vi "Pump Initialize Hardware References.vi"(8 "error in (no error)":errorcluster, 11 "Hardware Resources in":T1 {"Pump Info"."Direction" items=["CW", "CCW"]; "Pump Info"."Speed" format="%03.0f"}) -> (0 "error out":errorcluster, 3 "Hardware Resources out":T1 {"Pump Info"."Direction" items=["CW", "CCW"]; "Pump Info"."Speed" format="%03.0f"})   [LabVIEW 2020, in "Pump.lvlib"]
doc: "Initialize the hardware references."
uses:
  Pump.lvlib
  Pump Hardware Configuration.ctl
  support/Message Queue/Message Cluster.ctl
  <instrlib>/WM Pump/WM Pump.lvlib
  support/Message Queue/Message Queue.lvlib
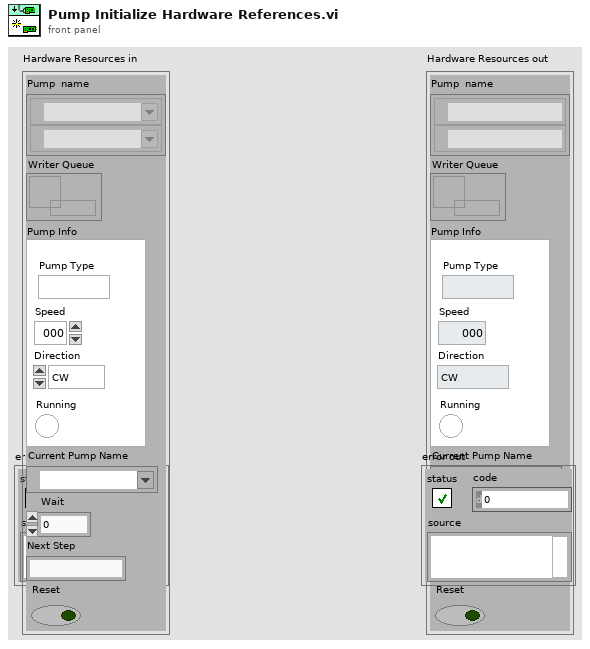
[diagram p1: front panel]
types:
  T1 = typedef "Pump.lvlib/Pump Hardware Configuration.ctl" = cluster{"Pump  name":refnum<visa-resource-name>[], "Writer Queue":refnum<queue>, "Pump Info":cluster{"Pump Type":string, "Speed":i32, "Direction":u16, "Running":bool}, "Current Pump Name":refnum<visa-resource-name>, "Wait":dbl, "Next Step":string, "Reset":bool}
  T2 = cluster{"Baud Rate":u32, "Parity":u16, "Data Bits":u16, "Stop Bits":u16, "Flow Control":u16}
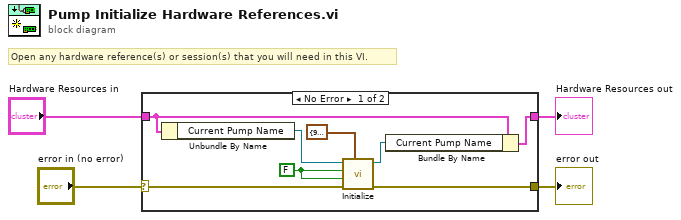
[diagram p0: block diagram]
diagram:
  # "Open any hardware reference(s) or session(s) that you will need in this VI."
  n1 = case shown="No Error" "error in (no error)" {
    selector: "error in (no error)" -> [w9 w13]
    tunnel: [w8 w13] -> w3
    tunnel: "Hardware Resources in" -> [w11 w14]
    tunnel: [w12 w14] -> w1
    frame No Error {
      w5 = FALSE ("ID Query (True)")
      n2 = Unbundle By Name(w11) -> ("Current Pump Name"=w10:refnum<visa-resource-name>)
      n3 = call <instrlib>:"Initialize.vi"("Serial Configuration"=T2 {"Baud Rate"=9600, "Parity"=0, "Data Bits"=8, "Stop Bits"=20, "Flow Control"=0}, "error in (no error)"=w9, "Reset (True)"=w5, "ID Query (True)"=w5, "VISA resource name"=w10) -> ("error out"=w8:errorcluster, "VISA resource name out"=w7:refnum<visa-resource-name>)  [unwired: 5 in]
      n4 = Bundle By Name(cluster=w11, "Current Pump Name"=w7) -> (w12:T1)
    }
    frame Error {
    }
  }
  "Hardware Resources out" <- w1
  "error out" <- w3
